vi "test mb.vi"() -> ()   [LabVIEW 2019]
uses:
  <vilib>/NI/Modbus Library/API/Wrapper/Create TCP Master.vi
  <vilib>/NI/Modbus Library/API/Master/Modbus Master.lvclass
  <vilib>/NI/Modbus Library/API/Wrapper/API Main.lvlib
panel:
  in  "Array":bool[](array[boolean])=[FALSE, FALSE, FALSE, FALSE, FALSE, FALSE, FALSE, FALSE, FALSE, FALSE, FALSE, FALSE, FALSE, FALSE, FALSE, FALSE]
  in  "address 2":u16
  in  "set":bool
  in  "register to write":u16
  in  "address":u16
  in  "stop":bool
  out "error out":errorcluster
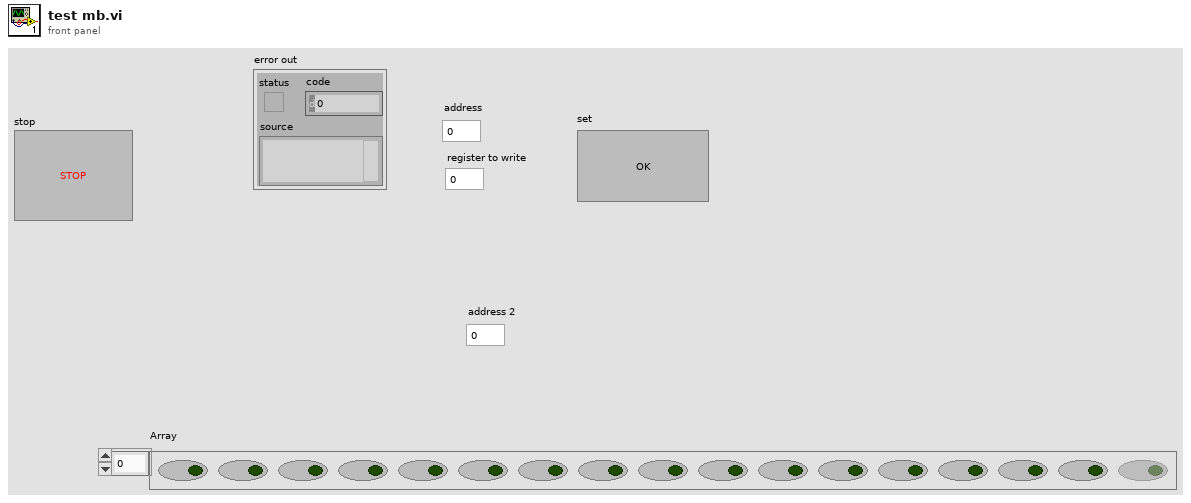
[diagram p1: front panel]
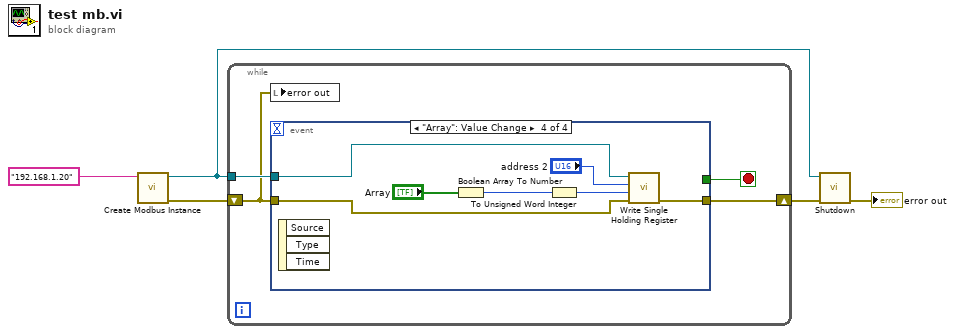
[diagram p0: block diagram]
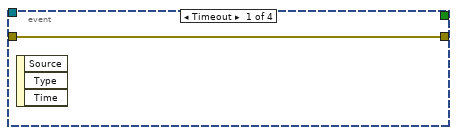
[diagram p2: hidden frame]
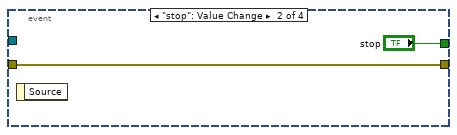
[diagram p3: hidden frame]
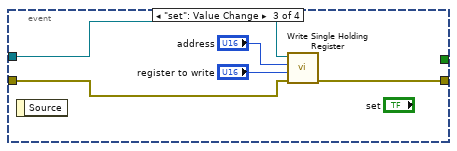
[diagram p4: hidden frame]
diagram:
  n1 = call-poly <vilib>:"Create Modbus Instance.vi"("address"="192.168.1.20") -> ("error out"=w3:errorcluster, "TCP master instance"=w1:refnum<class "Modbus Master.lvclass">)  [unwired: 9 in]
  n2 = while {
    shift-right: [w7] -> w2
    shift-left: w3 -> [w6]
    tunnel: w1 -> [w8]
    stop <- w9 stop-if-true
    n3 = local write "error out"(w6) -> ()
    n4 = event shown="[3] \"Array\": Value Change" {
      selector: _ -> [_ _ _ _]
      dyn-events: _ -> [_ _ _ _]
      timeout: _ -> [_ _ _ _]
      tunnel: [_ "stop" _ _] -> w9
      tunnel: w8 -> [_ _ w15 w23]
      tunnel: w6 -> [w10 w11 w14 w22]
      tunnel: [w10 w11 w13 w21] -> w7
      event Timeout {
        n5 = event-data() -> ()  [unwired: 1 in, 3 out]
      }
      event "stop": Value Change {
        n6 = event-data() -> ()  [unwired: 1 in, 1 out]
      }
      event "set": Value Change {
        n7 = event-data() -> ()  [unwired: 1 in, 1 out]
        n8 = call-dynamic "Write Single Holding Register.vi"("error in"=w14, "register to write"="register to write", "address"="address", "Modbus master in"=w15) -> ("error out"=w13:errorcluster)  [unwired: 6 in, 1 out]
      }
      event "Array": Value Change {
        n9 = event-data() -> ()  [unwired: 1 in, 3 out]
        n10 = Boolean Array To Number(Boolean array="Array") -> (number=w19:u32)
        n11 = To Unsigned Word Integer(number=w19) -> (unsigned 16bit integer=w18:u16)
        n12 = call-dynamic "Write Single Holding Register.vi"("error in"=w22, "register to write"=w18, "address"="address 2", "Modbus master in"=w23) -> ("error out"=w21:errorcluster)  [unwired: 6 in, 1 out]
      }
    }
  }
  n13 = call-dynamic "Shutdown.vi"("error in"=w2, "Modbus master in"=w1) -> ("error out"=→"error out":errorcluster)  [unwired: 9 in]
